vi "Trap Frequency AFG Control.vi"() -> ()   [LabVIEW 2012]
doc: "Shows how to generate a standard waveform."
uses:
  Public/Agilent 33XXX Series.lvlib
panel:
  in  "Slope":u16(ring) items=["Positive", "Negative"]
  in  "Trigger Source":u16(ring)=1 items=["Internal", "External", "Software (bus)"]
  in  "Waveform":u16(ring)=1 items=["DC", "Sine", "Square", "Triangle", "Ramp", "Pulse", "Noise", "Sinc", "Negative Ramp", "Exponential Rise", "Exponential Fall", "Cardiac"]
  in  "Enable Output":bool=TRUE
  in  "stop":bool
  in  "Burst Count":i32=10
  in  "Burst Mode":u16(ring)=1 items=["Triggered", "Gated"]
  in  "Frequency":dbl=1000.0
  in  "Serial Configuration":T1={"Baud Rate"=9600, "Parity"=0, "Data Bits"=8, "Flow Control"=4} {"Flow Control" items=["None", "XON/XOFF", "RTS/CTS", "XON/XOFF & RTS/CTS", "DTR/DSR", "XON/XOFF & DTR/DSR"]; "Data Bits" items=["7"=7, "8"=8]; "Parity" items=["None", "Odd", "Even", "Mark", "Space"]; "Baud Rate" items=["300"=300, "600"=600, "1200"=1200, "2400"=2400, "4800"=4800, "9600"=9600, "19200"=19200]}
  in  "Amplitude":dbl=1.0
  in  "VISA resource name":refnum<visa-resource-name>="GPIB0::5::INSTR"
  # "(c) 2005 - 2013 National Instruments.  ALL RIGHTS RESERVED."
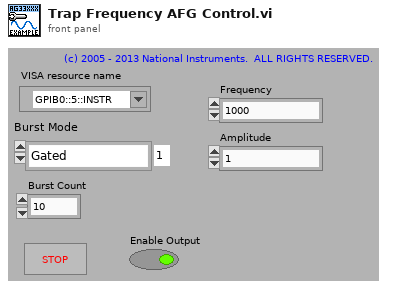
[diagram p1: front panel]
types:
  T1 = cluster{"Baud Rate":u32, "Parity":u16, "Data Bits":u16, "Flow Control":u16}
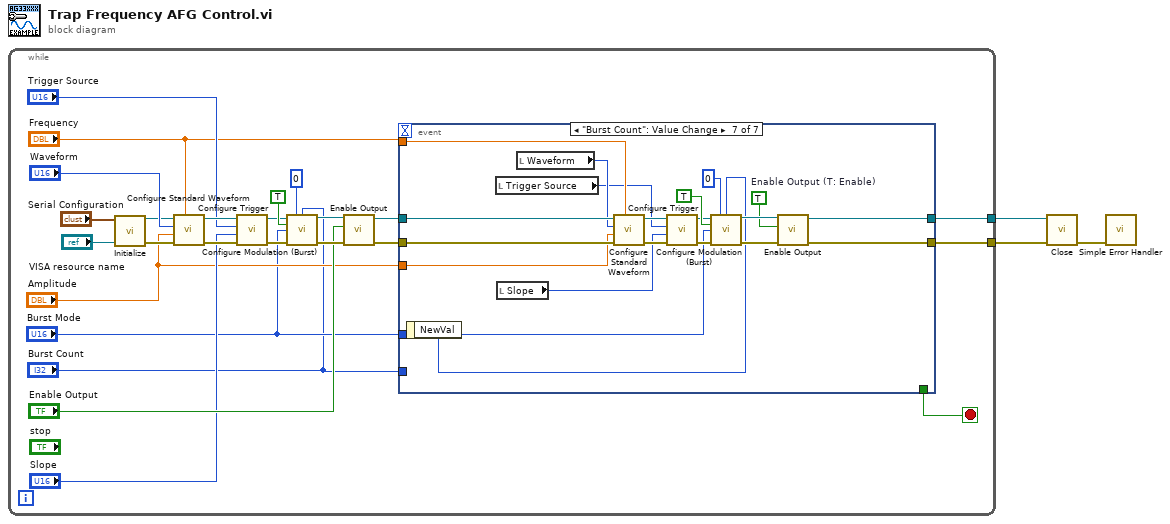
[diagram p0: block diagram]
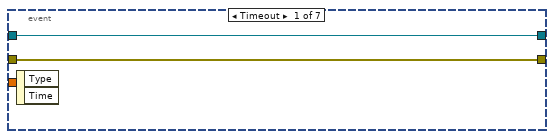
[diagram p2: hidden frame]
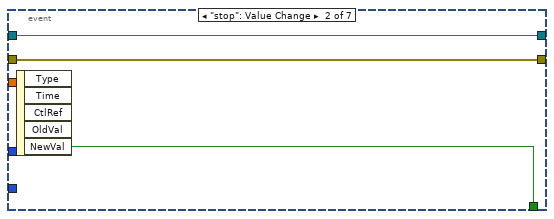
[diagram p3: hidden frame]
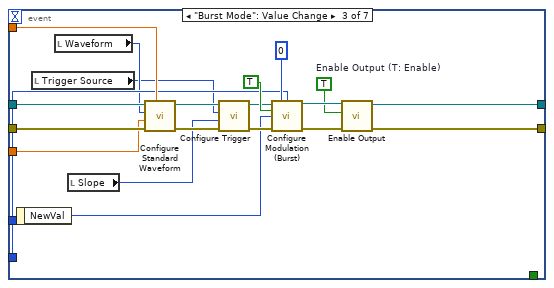
[diagram p4: hidden frame]
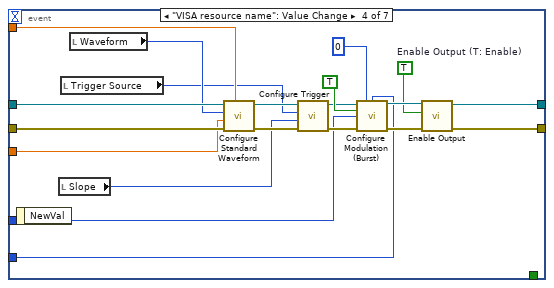
[diagram p5: hidden frame]
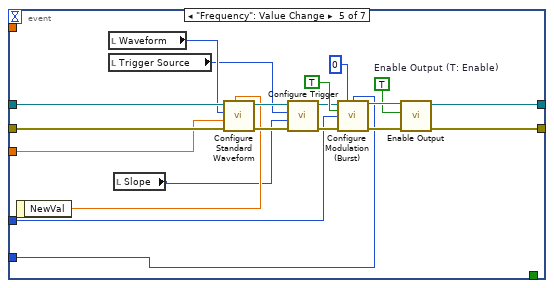
[diagram p6: hidden frame]
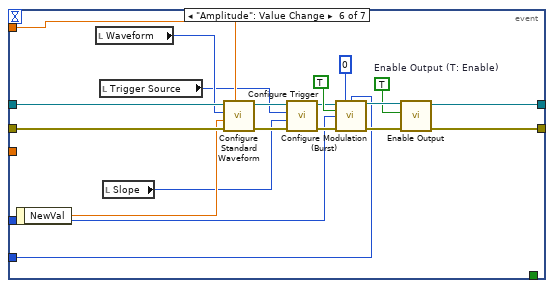
[diagram p7: hidden frame]
diagram:
  n1 = while {
    tunnel: [w26] -> w2
    tunnel: [w25] -> w1
    stop <- w24 stop-if-true
    n2 = call "Initialize.vi"("Serial Configuration"="Serial Configuration", "VISA resource name"="VISA resource name") -> ("error out"=w10:errorcluster, "VISA resource name out"=w11:refnum<visa-resource-name>)  [unwired: 8 in]
    n3 = call "Configure Standard Waveform.vi"("Frequency (1000 Hz)"="Frequency", "error in (no error)"=w10, "Amplitude (1)"="Amplitude", "Waveform Function (1: Sine)"="Waveform", "VISA resource name"=w11) -> ("error out"=w19:errorcluster, "VISA resource name out"=w18:refnum<visa-resource-name>)  [unwired: 5 in]
    n4 = call "Configure Trigger.vi"("error in (no error)"=w19, "Slope (0: Positive)"="Slope", "Trigger Source (0: Internal)"="Trigger Source", "VISA resource name"=w18) -> ("error out"=w17:errorcluster, "VISA resource name out"=w16:refnum<visa-resource-name>)  [unwired: 6 in]
    n5 = call "Configure Modulation (Burst).vi"("VISA resource name"=w16, "Burst Phase (0 deg)"=0, "Burst Count (1)"="Burst Count", "Enable Burst Modulation (T: Enable)"=TRUE ("Enable Burst"), "Burst Modulation Mode (0: Triggered)"="Burst Mode", "error in (no error)"=w17) -> ("VISA resource name out"=w21:refnum<visa-resource-name>, "error out"=w22:errorcluster)  [unwired: 8 in]
    n6 = call "Enable Output.vi"("error in (no error)"=w22, "Enable Output  (T: Enable)"="Enable Output", "VISA resource name"=w21) -> ("error out"=w4:errorcluster, "VISA resource name out"=w5:refnum<visa-resource-name>)  [unwired: 7 in]
    n7 = event shown="[6] \"Burst Count \": Value Change" {
      selector: _ -> [_ _ _ _ _ _ _]
      dyn-events: _ -> [_ _ _ _ _ _ _]
      timeout: _ -> [_ _ _ _ _ _ _]
      tunnel: w5 -> [w30 w32 w45 w65 w85 w105 w125]
      tunnel: w4 -> [w29 w31 w44 w64 w84 w104 w124]
      tunnel: "Amplitude" -> [_ _ w43 w63 w83 _ w118]
      tunnel: "Frequency" -> [_ _ w42 w62 _ w98 w119]
      tunnel: "Burst Count" -> [_ _ w39 w60 w77 w102 _]
      tunnel: [w30 w32 w38 w59 w81 w101 w122] -> w26
      tunnel: [w29 w31 w37 w58 w80 w100 w121] -> w25
      tunnel: [_ w33 _ _ _ _ _] -> w24
      tunnel: "Burst Mode" -> [_ _ _ w57 w79 w95 w120]
      event Timeout {
        n8 = event-data() -> ()  [unwired: 1 in, 2 out]
      }
      event "stop": Value Change {
        n9 = event-data() -> ("NewVal"=w33:bool)  [unwired: 1 in, 4 out]
      }
      event "Burst Mode": Value Change {
        w50 = TRUE  # Enable Output (T: Enable)
        n10 = event-data() -> ("NewVal"=w41:u16)  [unwired: 1 in]
        n11 = local read "Trigger Source"() -> (w35:u16)
        n12 = local read "Waveform"() -> (w36:u16)
        n13 = local read "Slope"() -> (w34:u16)
        n14 = call "Configure Standard Waveform.vi"("Frequency (1000 Hz)"=w42, "error in (no error)"=w44, "Amplitude (1)"=w43, "Waveform Function (1: Sine)"=w36, "VISA resource name"=w45) -> ("error out"=w49:errorcluster, "VISA resource name out"=w48:refnum<visa-resource-name>)  [unwired: 5 in]
        n15 = call "Configure Trigger.vi"("error in (no error)"=w49, "Slope (0: Positive)"=w34, "Trigger Source (0: Internal)"=w35, "VISA resource name"=w48) -> ("error out"=w47:errorcluster, "VISA resource name out"=w46:refnum<visa-resource-name>)  [unwired: 6 in]
        n16 = call "Configure Modulation (Burst).vi"("VISA resource name"=w46, "Burst Phase (0 deg)"=0, "Burst Count (1)"=w39, "Enable Burst Modulation (T: Enable)"=TRUE ("Enable Burst"), "Burst Modulation Mode (0: Triggered)"=w41, "error in (no error)"=w47) -> ("VISA resource name out"=w51:refnum<visa-resource-name>, "error out"=w52:errorcluster)  [unwired: 8 in]
        n17 = call "Enable Output.vi"("error in (no error)"=w52, "Enable Output  (T: Enable)"=w50, "VISA resource name"=w51) -> ("error out"=w37:errorcluster, "VISA resource name out"=w38:refnum<visa-resource-name>)  [unwired: 7 in]
      }
      event "VISA resource name": Value Change {
        w70 = TRUE  # Enable Output (T: Enable)
        n18 = event-data() -> ()  [unwired: 1 in, 1 out]
        n19 = local read "Slope"() -> (w54:u16)
        n20 = local read "Trigger Source"() -> (w55:u16)
        n21 = local read "Waveform"() -> (w56:u16)
        n22 = call "Configure Standard Waveform.vi"("Frequency (1000 Hz)"=w62, "error in (no error)"=w64, "Amplitude (1)"=w63, "Waveform Function (1: Sine)"=w56, "VISA resource name"=w65) -> ("error out"=w69:errorcluster, "VISA resource name out"=w68:refnum<visa-resource-name>)  [unwired: 5 in]
        n23 = call "Configure Trigger.vi"("error in (no error)"=w69, "Slope (0: Positive)"=w54, "Trigger Source (0: Internal)"=w55, "VISA resource name"=w68) -> ("error out"=w67:errorcluster, "VISA resource name out"=w66:refnum<visa-resource-name>)  [unwired: 6 in]
        n24 = call "Configure Modulation (Burst).vi"("VISA resource name"=w66, "Burst Phase (0 deg)"=0, "Burst Count (1)"=w60, "Enable Burst Modulation (T: Enable)"=TRUE ("Enable Burst"), "Burst Modulation Mode (0: Triggered)"=w57, "error in (no error)"=w67) -> ("VISA resource name out"=w71:refnum<visa-resource-name>, "error out"=w72:errorcluster)  [unwired: 8 in]
        n25 = call "Enable Output.vi"("error in (no error)"=w72, "Enable Output  (T: Enable)"=w70, "VISA resource name"=w71) -> ("error out"=w58:errorcluster, "VISA resource name out"=w59:refnum<visa-resource-name>)  [unwired: 7 in]
      }
      event "Frequency": Value Change {
        w90 = TRUE  # Enable Output (T: Enable)
        n26 = event-data() -> ("NewVal"=w78:dbl)  [unwired: 1 in]
        n27 = local read "Waveform"() -> (w76:u16)
        n28 = local read "Trigger Source"() -> (w75:u16)
        n29 = local read "Slope"() -> (w74:u16)
        n30 = call "Configure Standard Waveform.vi"("Frequency (1000 Hz)"=w78, "error in (no error)"=w84, "Amplitude (1)"=w83, "Waveform Function (1: Sine)"=w76, "VISA resource name"=w85) -> ("error out"=w89:errorcluster, "VISA resource name out"=w88:refnum<visa-resource-name>)  [unwired: 5 in]
        n31 = call "Configure Trigger.vi"("error in (no error)"=w89, "Slope (0: Positive)"=w74, "Trigger Source (0: Internal)"=w75, "VISA resource name"=w88) -> ("error out"=w87:errorcluster, "VISA resource name out"=w86:refnum<visa-resource-name>)  [unwired: 6 in]
        n32 = call "Configure Modulation (Burst).vi"("VISA resource name"=w86, "Burst Phase (0 deg)"=0, "Burst Count (1)"=w77, "Enable Burst Modulation (T: Enable)"=TRUE ("Enable Burst"), "Burst Modulation Mode (0: Triggered)"=w79, "error in (no error)"=w87) -> ("VISA resource name out"=w91:refnum<visa-resource-name>, "error out"=w92:errorcluster)  [unwired: 8 in]
        n33 = call "Enable Output.vi"("error in (no error)"=w92, "Enable Output  (T: Enable)"=w90, "VISA resource name"=w91) -> ("error out"=w80:errorcluster, "VISA resource name out"=w81:refnum<visa-resource-name>)  [unwired: 7 in]
      }
      event "Amplitude": Value Change {
        w110 = TRUE  # Enable Output (T: Enable)
        n34 = event-data() -> ("NewVal"=w99:dbl)  [unwired: 1 in]
        n35 = local read "Waveform"() -> (w97:u16)
        n36 = local read "Trigger Source"() -> (w96:u16)
        n37 = local read "Slope"() -> (w94:u16)
        n38 = call "Configure Standard Waveform.vi"("Frequency (1000 Hz)"=w98, "error in (no error)"=w104, "Amplitude (1)"=w99, "Waveform Function (1: Sine)"=w97, "VISA resource name"=w105) -> ("error out"=w109:errorcluster, "VISA resource name out"=w108:refnum<visa-resource-name>)  [unwired: 5 in]
        n39 = call "Configure Trigger.vi"("error in (no error)"=w109, "Slope (0: Positive)"=w94, "Trigger Source (0: Internal)"=w96, "VISA resource name"=w108) -> ("error out"=w107:errorcluster, "VISA resource name out"=w106:refnum<visa-resource-name>)  [unwired: 6 in]
        n40 = call "Configure Modulation (Burst).vi"("VISA resource name"=w106, "Burst Phase (0 deg)"=0, "Burst Count (1)"=w102, "Enable Burst Modulation (T: Enable)"=TRUE ("Enable Burst"), "Burst Modulation Mode (0: Triggered)"=w95, "error in (no error)"=w107) -> ("VISA resource name out"=w111:refnum<visa-resource-name>, "error out"=w112:errorcluster)  [unwired: 8 in]
        n41 = call "Enable Output.vi"("error in (no error)"=w112, "Enable Output  (T: Enable)"=w110, "VISA resource name"=w111) -> ("error out"=w100:errorcluster, "VISA resource name out"=w101:refnum<visa-resource-name>)  [unwired: 7 in]
      }
      event "Burst Count": Value Change {
        w130 = TRUE  # Enable Output (T: Enable)
        n42 = event-data() -> ("NewVal"=w117:i32)  [unwired: 1 in]
        n43 = local read "Trigger Source"() -> (w115:u16)
        n44 = local read "Slope"() -> (w114:u16)
        n45 = local read "Waveform"() -> (w116:u16)
        n46 = call "Configure Standard Waveform.vi"("Frequency (1000 Hz)"=w119, "error in (no error)"=w124, "Amplitude (1)"=w118, "Waveform Function (1: Sine)"=w116, "VISA resource name"=w125) -> ("error out"=w129:errorcluster, "VISA resource name out"=w128:refnum<visa-resource-name>)  [unwired: 5 in]
        n47 = call "Configure Trigger.vi"("error in (no error)"=w129, "Slope (0: Positive)"=w114, "Trigger Source (0: Internal)"=w115, "VISA resource name"=w128) -> ("error out"=w127:errorcluster, "VISA resource name out"=w126:refnum<visa-resource-name>)  [unwired: 6 in]
        n48 = call "Configure Modulation (Burst).vi"("VISA resource name"=w126, "Burst Phase (0 deg)"=0, "Burst Count (1)"=w117, "Enable Burst Modulation (T: Enable)"=TRUE ("Enable Burst"), "Burst Modulation Mode (0: Triggered)"=w120, "error in (no error)"=w127) -> ("VISA resource name out"=w131:refnum<visa-resource-name>, "error out"=w132:errorcluster)  [unwired: 8 in]
        n49 = call "Enable Output.vi"("error in (no error)"=w132, "Enable Output  (T: Enable)"=w130, "VISA resource name"=w131) -> ("error out"=w121:errorcluster, "VISA resource name out"=w122:refnum<visa-resource-name>)  [unwired: 7 in]
      }
    }
  }
  n50 = call "Close.vi"("error in (no error)"=w1, "VISA resource name"=w2) -> ("error out"=w3:errorcluster)  [unwired: 9 in]
  n51 = call <vilib>:"Simple Error Handler.vi"("error in (no error)"=w3) -> ()  [unwired: 4 in, 5 out]
